vi "Create File.vi"(8 "error in":errorcluster, 11 "Root Path":path) -> (0 "error out":errorcluster, 1 "File Path Out":path, 3 "Refnum Out":refnum<file>)   [LabVIEW 2021]
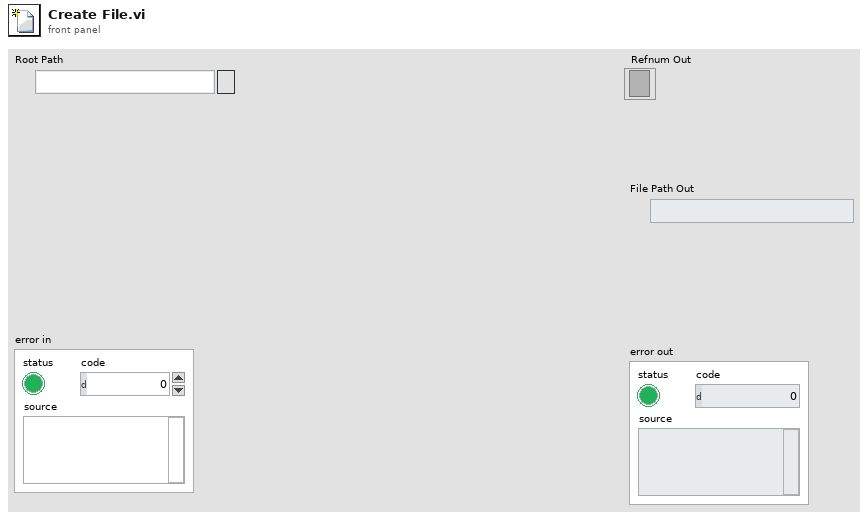
[diagram p1: front panel]
types:
  T1 = enum16{"open", "replace", "create", "open or create", "replace or create", "replace or create with confirmation"}
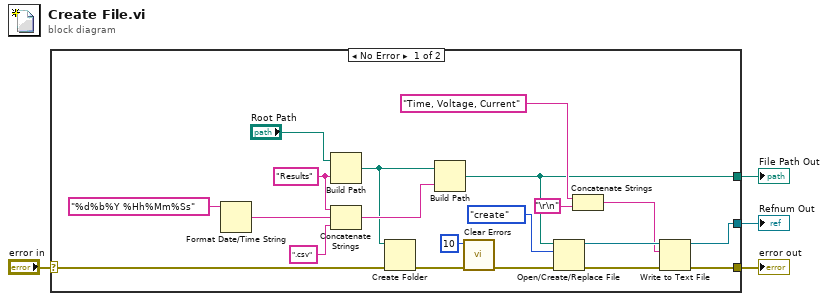
[diagram p0: block diagram]
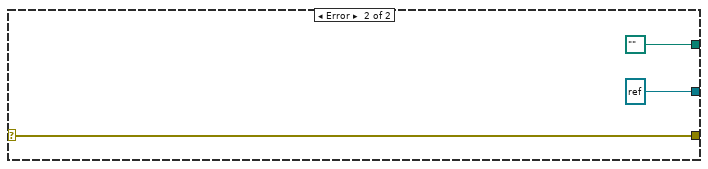
[diagram p2: hidden frame]
diagram:
  n1 = case shown="No Error" "error in" {
    selector: "error in" -> [w7 w27]
    tunnel: [w16 w27] -> w3
    tunnel: [w12 refnum<file> refnum ("refnum out")] -> w2
    tunnel: [w11 path "" ("appended path")] -> w1
    frame No Error {
      w21 = "Results" ("string")
      n2 = Format Date/Time String(time format string (%c)="%d%b%Y %Hh%Mm%Ss") -> (date/time string=w23:string)  [unwired: 2 in]
      n3 = Build Path(base path="Root Path", name or relative path=w21) -> (appended path=w8:path)
      n4 = Concatenate Strings "Concatenate Strings"(w21, w23, ".csv" ("string")) -> (w20:string)
      n5 = Create Folder(path (use dialog)=w8, error in=w7) -> (error out=w6:errorcluster)  [unwired: 1 in, 2 out]
      n6 = Build Path(base path=w8, name or relative path=w20) -> (appended path=w11:path)
      n7 = call <vilib>:"Clear Errors.vi"("error in (no error)"=w6, "specific error code to clear (0: all)"=10) -> ("error out"=w5:errorcluster)  [unwired: 4 in, 1 out]
      n8 = Open/Create/Replace File(file path (use dialog)=w11, error in=w5, operation (0:open)=T1."create") -> (refnum out=w18:refnum<file>, error out=w17:errorcluster)  [unwired: 3 in, 1 out]
      n9 = Concatenate Strings "Concatenate Strings"("Time, Voltage, Current" ("string"), "\r\n") -> (w13:string)
      n10 = Write to Text File(file (use dialog)=w18, text=w13, error in=w17) -> (refnum out=w12:refnum<file>, error out=w16:errorcluster)  [unwired: 1 in, 1 out]
    }
    frame Error {
    }
  }
  "error out" <- w3
  "File Path Out" <- w1
  "Refnum Out" <- w2
